vi "Parse and Log Group Data.vi"(8 "error in (no error)":errorcluster, 10 "Data":variant, 11 "Report Generator in":refnum<class "Report Generator.lvclass">) -> (0 "error out":errorcluster, 3 "Report Generator out":refnum<class "Report Generator.lvclass">)   [LabVIEW 2023, in "Report Generator.lvlib" / "Report Generator.lvclass"]
doc: "Enforce Group Properties formatting\nThen call Write Group Properties.\nExpects variant to contain:\n<b>String: Group</b> - empty string is a legal value for test properties\n<b>String:Array Property Names</b> Array of string names for property names to be set\n<b>Variant:Array </b> Any legal loggable value for a property"
uses:
  Library/Report Generator.lvclass
  Library/Report Generator.lvclass/Report Generator.ctl
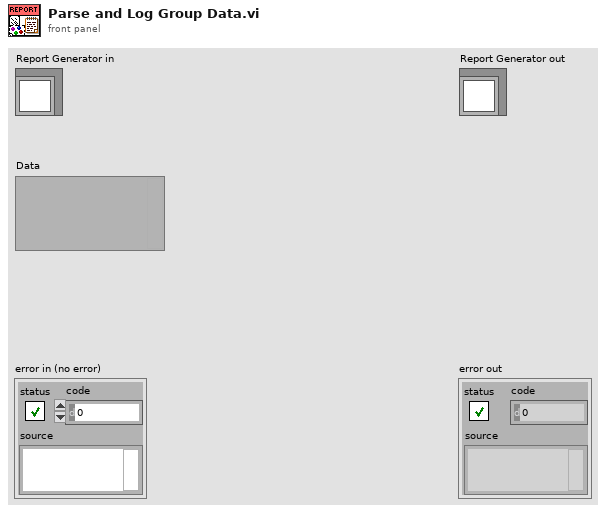
[diagram p1: front panel]
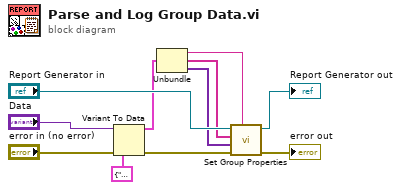
[diagram p0: block diagram]
diagram:
  n1 = Variant To Data(error in="error in (no error)", type=cluster{string, string[], variant[]} {"", [], []}, Variant="Data") -> (data=w7:cluster{string, string[], variant[]}, error out=w1:errorcluster)
  n2 = Unbundle(w7) -> (w6:string, w5:string[], w4:variant[])
  n3 = call-dynamic "Set Group Properties.vi"("Group"=w6, "error in (no error)"=w1, "Values"=w4, "Parameters"=w5, "Report Generator in"="Report Generator in") -> ("error out"=→"error out":errorcluster, "Report Generator out"=→"Report Generator out":refnum<class "Report Generator.lvclass">)  [unwired: 5 in]
